vi "TerminalWrite.vi"(8 "error in":errorcluster, 10 "string":string, 11 "TerminalIn":T1) -> (0 "error out":errorcluster, 3 "TerminalOut":T1)   [LabVIEW 2021, in "LibDan.lvlib"]
uses:
  LibDan.lvlib
  TerminalDef.ctl
  <vilib>/Utility/config.llb/Config Data RefNum.ctl
  <vilib>/Utility/config.llb/NI_LVConfig.lvlib
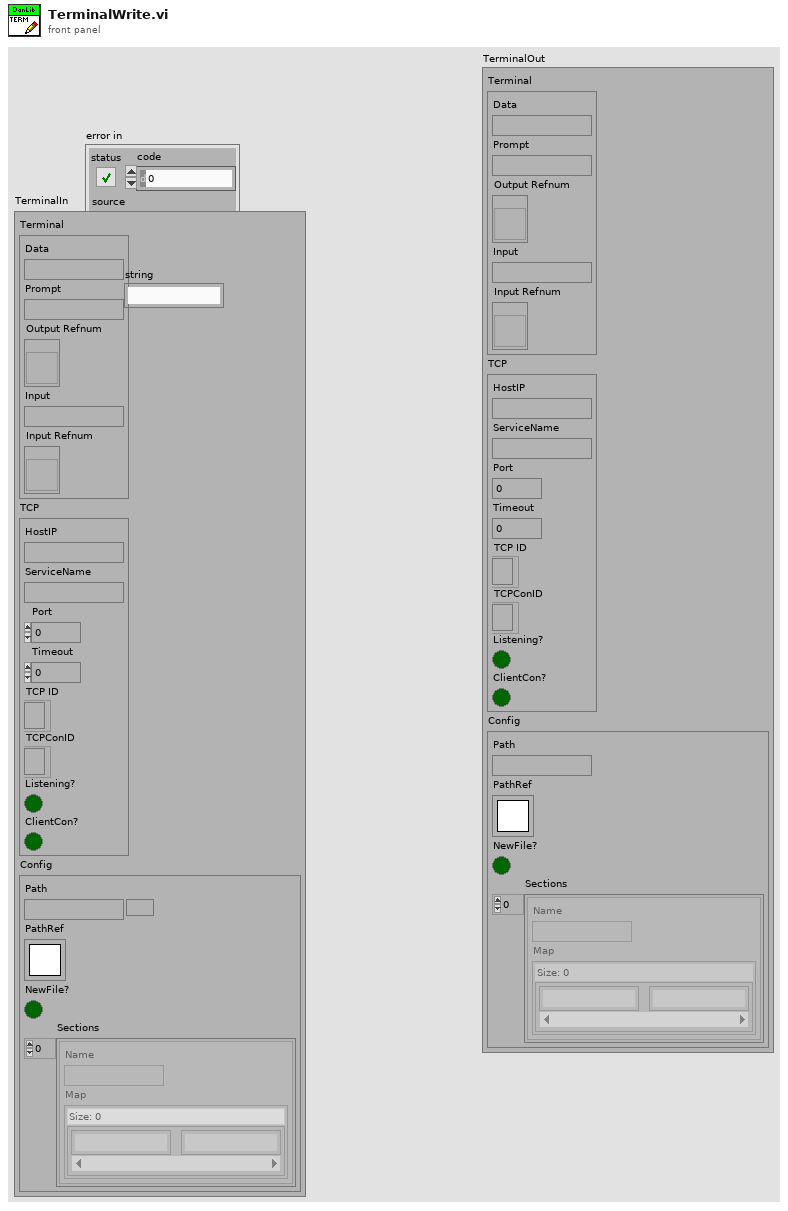
[diagram p1: front panel]
types:
  T1 = typedef "LibDan.lvlib/TerminalDef.ctl" = cluster{"Terminal":cluster{"Data":string, "Prompt":string, "Output Refnum":refnum<vi>, "Input":string, "Input Refnum":refnum<vi>}, "TCP":cluster{"HostIP":string, "ServiceName":string, "Port":u16, "Timeout":i32, "TCP ID":refnum<k5>, "TCPConID":refnum<k5>, "Listening?":bool, "ClientCon?":bool}, "Config":cluster{"Path":path, "PathRef":T2, "NewFile?":bool, "Sections":cluster{"Name":string, "Map":map{string, string}}[]}}
  T2 = typedef "NI_LVConfig.lvlib/Config Data RefNum.ctl" = refnum<k1>
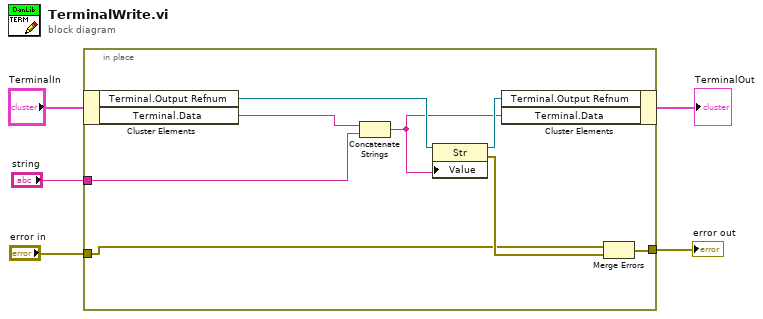
[diagram p0: block diagram]
diagram:
  n1 = in-place {
    in-place-border: "error in" -> [w6]
    in-place-border: [w8] -> w3
    in-place-border: "string" -> [w9]
    n2 = in-place-cluster #1("TerminalIn") -> ("Terminal.Output Refnum"=w13:refnum<vi>, "Terminal.Data"=w11:string)
    n3 = Concatenate Strings(w11, w9) -> (w10:string)
    n4 = property class="Str"(reference=w13, "Value"=w10) -> (reference out=w12:refnum<vi>, error out=w7:errorcluster)  [unwired: 1 in]
    n5 = in-place-cluster #1("Terminal.Output Refnum"=w12, "Terminal.Data"=w10) -> (→"TerminalOut":T1)
    n6 = Merge Errors(w6, w7) -> (w8:errorcluster)
  }
  "error out" <- w3
